vi "set_continuous_samples.vi"(8 "error in (no error)":errorcluster, 10 "continuous samples":i32, 11 "GenericWriteSignals.lvclass in":refnum<class "SignalWriterMH110203USBStepperMotor.lvclass">) -> (0 "error out":errorcluster, 3 "GenericWriteSignals.lvclass out":refnum<class "SignalWriterMH110203USBStepperMotor.lvclass">)   [LabVIEW 2010, in "SignalWriterMH110203USBStepperMotor.lvclass"]
uses:
  SignalWriterMH110203USBStepperMotor.lvclass
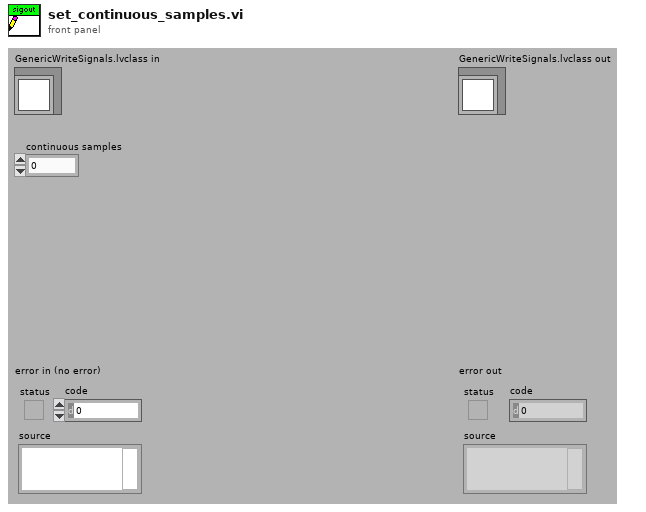
[diagram p1: front panel]
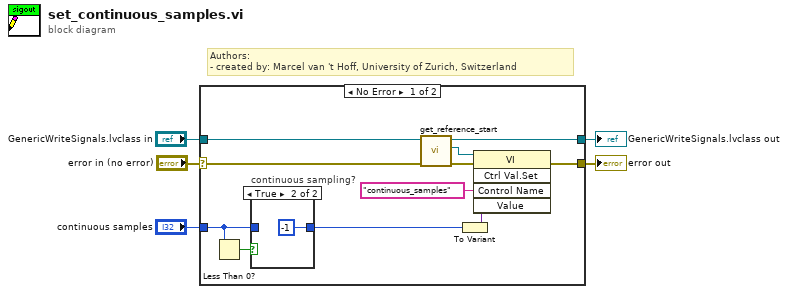
[diagram p0: block diagram]
diagram:
  # "Authors: \n- created by: Marcel van 't Hoff, University of Zurich, Switzerland"
  n1 = case shown="No Error" "error in (no error)" {
    selector: "error in (no error)" -> [w10 w20]
    tunnel: [w9 w20] -> w2
    tunnel: "GenericWriteSignals.lvclass in" -> [w12 w19]
    tunnel: "continuous samples" -> [w6 _]
    tunnel: [w11 w19] -> w3
    frame No Error {
      n2 = Less Than 0?(x=w6) -> (x < 0?=w8:bool)
      n3 = case "continuous sampling?" shown="True" w8 {
        tunnel: [w17 -1 ("continuous samples")] -> w7
        tunnel: w6 -> [w17 _]
        frame False {
        }
        frame True {
        }
      }
      n4 = call-dynamic "get_reference_start.vi"("error in (no error)"=w10, "SignalWriterMH110203USBStepperMotor in"=w12) -> ("error out"=w15:errorcluster, "vi reference"=w16:refnum<vi>, "SignalWriterMH110203USBStepperMotor out"=w11:refnum<class "SignalWriterMH110203USBStepperMotor.lvclass">)  [unwired: 7 in]
      n5 = To Variant(anything=w7) -> (Variant=w14:variant)
      n6 = invoke class="VI" method="Ctrl Val.Set"(reference=w16, error in=w15, "Control Name"="continuous_samples", "Value"=w14) -> (error out=w9:errorcluster)  [unwired: 1 in, 4 out]
    }
    frame Error {
    }
  }
  "error out" <- w2
  "GenericWriteSignals.lvclass out" <- w3
